vi "ConvertToData.vi"(8 "error in (no error)":errorcluster, 11 "Mediciones":string[][](array[string])) -> (0 "error out":errorcluster, 1 "Array Parsed Expression Out":T2[](array[typedef]), 2 "Dcte":sgl[](array[numeric]), 3 "Kcte":sgl[](array[numeric]), 4 "Conf. Gral.":T1)   [LabVIEW 2014, in "MathLoop.lvlib"]
doc: "Convierte los datos de las tablas de Mediciones (2D array) en Ctes, Dimensiones y arma el Array Parsed Expression."
uses:
  MathLoop.lvlib
  TypeDefs/ParsedExpression.ctl
  TypeDefs/typeMed.ctl
  TypeDefs/Conf. Gral.ctl
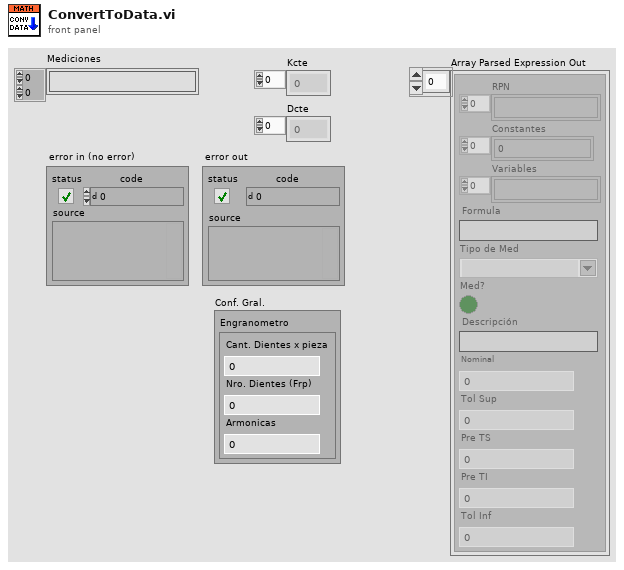
[diagram p1: front panel]
types:
  T1 = typedef "MathLoop.lvlib/Conf. Gral.ctl" = cluster{"Engranometro":cluster{"Cant. Dientes x pieza":i32, "Nro. Dientes (Frp)":i32, "Armonicas":i32}}
  T2 = typedef "MathLoop.lvlib/ParsedExpression.ctl" = cluster{"RPN ":string[], "Constantes":sgl[], "Variables":string[], "Formula":string, "Tipo de Med":T3, "Med?":bool, "Descripción":string, "Nominal":sgl, "Tol Sup":sgl, "Pre TS":sgl, "Pre TI":sgl, "Tol Inf":sgl}
  T3 = typedef "MathLoop.lvlib/typeMed.ctl" = string
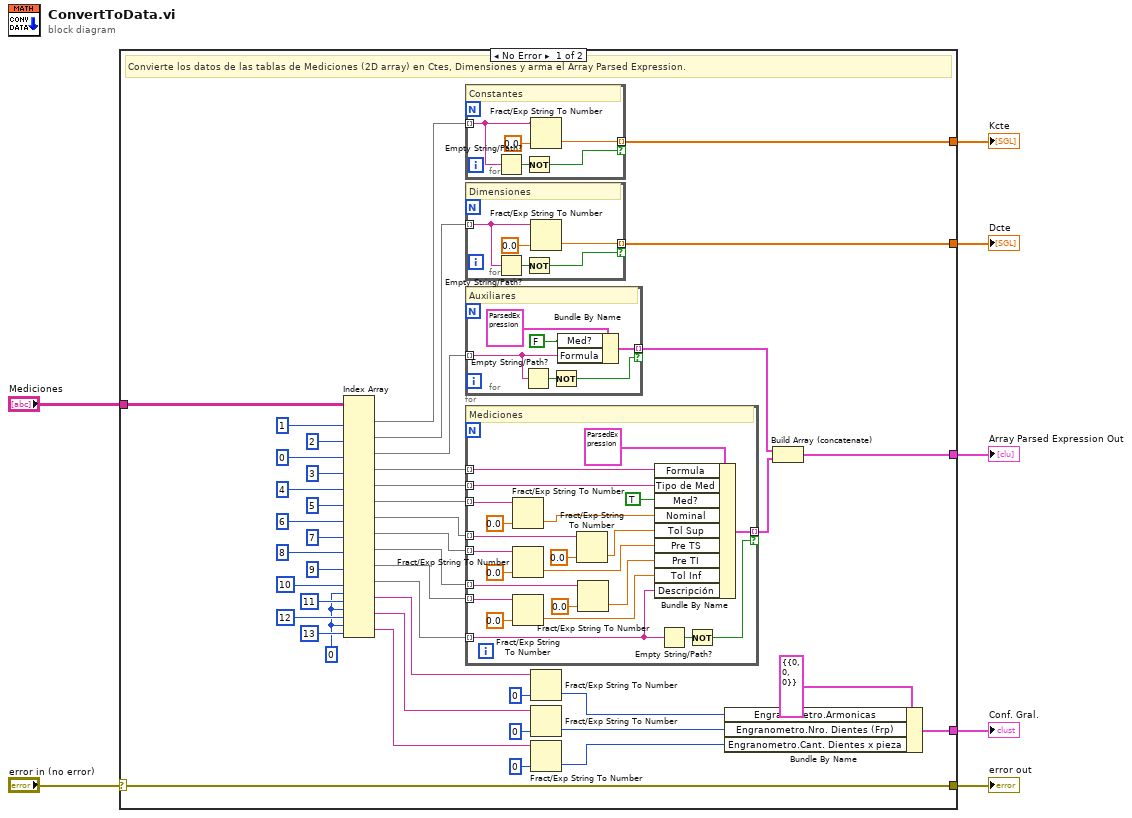
[diagram p0: block diagram]
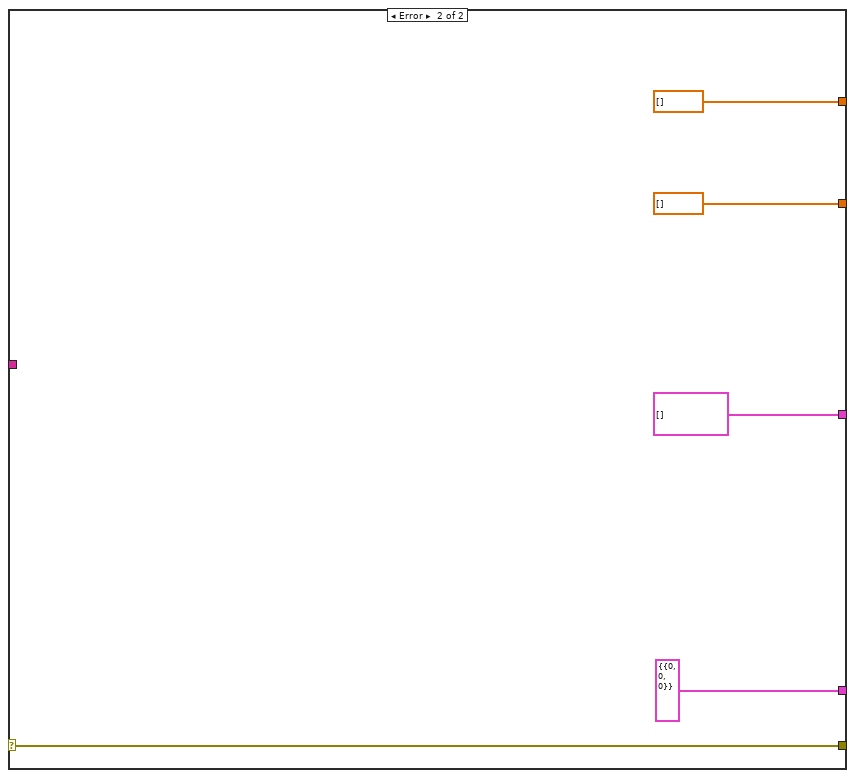
[diagram p2: hidden frame]
diagram:
  n1 = case shown="No Error" "error in (no error)" {
    selector: "error in (no error)" -> [w24 w95]
    tunnel: "Mediciones" -> [w23 _]
    tunnel: [w27 sgl[] []] -> w3
    tunnel: [w26 sgl[] []] -> w4
    tunnel: [w25 T2[] []] -> w2
    tunnel: [w24 w95] -> w5
    tunnel: [w11 T1 {"Engranometro"={"Cant. Dientes x pieza"=0, "Nro. Dientes (Frp)"=0, "Armonicas"=0}} ("Conf. Gral.")] -> w1
    frame No Error {
      w13 = 0 ("disabled index (col)")
      # "Convierte los datos de las tablas de Mediciones (2D array) en Ctes, Dimensiones y arma el Array Parsed Expression."
      n2 = Index Array(array=w23, index (col) #1=1 ("disabled index (col)"), index (col) #2=2 ("disabled index (col)"), index (col) #3=0 ("disabled index (col)"), index (col) #4=3 ("disabled index (col)"), index (col) #5=4 ("disabled index (col)"), index (col) #6=5 ("disabled index (col)"), index (col) #7=6 ("disabled index (col)"), index (col) #8=7 ("disabled index (col)"), index (col) #9=8 ("disabled index (col)"), index (col) #10=9 ("disabled index (col)"), index (col) #11=10 ("disabled index (col)"), index (row) #12=w13, index (col) #12=11 ("disabled index (col)"), index (row) #13=w13, index (col) #13=12 ("disabled index (col)"), index (row) #14=w13, index (col) #14=13 ("disabled index (col)")) -> (element #1=w32:string[], element #2=w33:string[], element #3=w42:string[], element #4=w41:string[], element #5=w40:string[], element #6=w39:string[], element #7=w38:string[], element #8=w37:string[], element #9=w36:string[], element #10=w35:string[], element #11=w34:string[], element #12=w19:string, element #13=w18:string, element #14=w17:string)  [unwired: 11 in]
      n3 = for {
        tunnel: w32 -> [w53] mode=indexing
        tunnel: [w52] -> w26 mode=indexing if=w55
        # "Constantes"
        n4 = Empty String/Path?(string/path=w53) -> (empty?=w56:bool)
        n5 = Not(x=w56) -> (.not. x?=w55:bool)
        n6 = Fract/Exp String To Number(string=w53, default (0 dbl)=sgl 0.0 ("default (0 DBL)")) -> (number=w52:sgl)  [unwired: 2 in, 1 out]
      }
      n7 = for {
        tunnel: w33 -> [w58] mode=indexing
        tunnel: [w57] -> w27 mode=indexing if=w60
        # "Dimensiones"
        n8 = Empty String/Path?(string/path=w58) -> (empty?=w61:bool)
        n9 = Not(x=w61) -> (.not. x?=w60:bool)
        n10 = Fract/Exp String To Number(string=w58, default (0 dbl)=sgl 0.0 ("default (0 DBL)")) -> (number=w57:sgl)  [unwired: 2 in, 1 out]
      }
      n11 = for {
        tunnel: w42 -> [w63] mode=indexing
        tunnel: [w65] -> w29 mode=indexing if=w66
        # "Auxiliares"
        n12 = Empty String/Path?(string/path=w63) -> (empty?=w67:bool)
        n13 = Not(x=w67) -> (.not. x?=w66:bool)
        n14 = Bundle By Name(cluster=T2 {"RPN "=[], "Constantes"=[], "Variables"=[], "Formula"="", "Tipo de Med"="", "Med?"=FALSE, "Descripción"="", "Nominal"=0.0, "Tol Sup"=0.0, "Pre TS"=0.0, "Pre TI"=0.0, "Tol Inf"=0.0} ("Parsed Expression"), "Med?"=FALSE, "Formula"=w63) -> (w65:T2)
      }
      n15 = for {
        tunnel: w41 -> [w74] mode=indexing
        tunnel: [w79] -> w28 mode=indexing if=w89
        tunnel: w40 -> [w73] mode=indexing
        tunnel: w39 -> [w84] mode=indexing
        tunnel: w38 -> [w83] mode=indexing
        tunnel: w37 -> [w82] mode=indexing
        tunnel: w36 -> [w81] mode=indexing
        tunnel: w35 -> [w80] mode=indexing
        tunnel: w34 -> [w77] mode=indexing
        # "Mediciones"
        n16 = Fract/Exp String To Number(string=w84, default (0 dbl)=sgl 0.0 ("default (0 DBL)")) -> (number=w71:sgl)  [unwired: 2 in, 1 out]
        n17 = Fract/Exp String To Number(string=w82, default (0 dbl)=sgl 0.0 ("default (0 DBL)")) -> (number=w69:sgl)  [unwired: 2 in, 1 out]
        n18 = Fract/Exp String To Number(string=w80, default (0 dbl)=sgl 0.0 ("default (0 DBL)")) -> (number=w76:sgl)  [unwired: 2 in, 1 out]
        n19 = Fract/Exp String To Number(string=w83, default (0 dbl)=sgl 0.0 ("default (0 DBL)")) -> (number=w70:sgl)  [unwired: 2 in, 1 out]
        n20 = Fract/Exp String To Number(string=w81, default (0 dbl)=sgl 0.0 ("default (0 DBL)")) -> (number=w68:sgl)  [unwired: 2 in, 1 out]
        n21 = Bundle By Name(cluster=T2 {"RPN "=[], "Constantes"=[], "Variables"=[], "Formula"="", "Tipo de Med"="", "Med?"=FALSE, "Descripción"="", "Nominal"=0.0, "Tol Sup"=0.0, "Pre TS"=0.0, "Pre TI"=0.0, "Tol Inf"=0.0} ("Parsed Expression Out"), "Formula"=w74, "Tipo de Med"=w73, "Med?"=TRUE, "Nominal"=w71, "Tol Sup"=w70, "Pre TS"=w69, "Pre TI"=w68, "Tol Inf"=w76, "Descripción"=w77) -> (w79:T2)
        n22 = Empty String/Path?(string/path=w77) -> (empty?=w90:bool)
        n23 = Not(x=w90) -> (.not. x?=w89:bool)
      }
      n24 = Fract/Exp String To Number(string=w19, default (0 dbl)=0 ("default (0 DBL)")) -> (number=w10:i32)  [unwired: 2 in, 1 out]
      n25 = Fract/Exp String To Number(string=w18, default (0 dbl)=0 ("default (0 DBL)")) -> (number=w9:i32)  [unwired: 2 in, 1 out]
      n26 = Fract/Exp String To Number(string=w17, default (0 dbl)=0 ("default (0 DBL)")) -> (number=w8:i32)  [unwired: 2 in, 1 out]
      n27 = Bundle By Name(cluster=T1 {"Engranometro"={"Cant. Dientes x pieza"=0, "Nro. Dientes (Frp)"=0, "Armonicas"=0}} ("Conf. Gral."), "Engranometro.Armonicas"=w10, "Engranometro.Nro. Dientes (Frp)"=w9, "Engranometro.Cant. Dientes x pieza"=w8) -> (w11:T1)
      n28 = Build Array (concatenate)(w29, w28) -> (w25:T2[])
    }
    frame Error {
    }
  }
  "error out" <- w5
  "Kcte" <- w4
  "Dcte" <- w3
  "Array Parsed Expression Out" <- w2
  "Conf. Gral." <- w1
